vi "ErrorToJSONString.vi"(8 "error in (no error)":errorcluster, 11 "problemJSON":string) -> (0 "error out":errorcluster, 3 "JSON Error string":string)   [LabVIEW 2013]
doc: "Converts an error code into a JSON object, optionally included a properly-quoted copy of the JSON that triggered it. Does not clear the error."
uses:
  <vilib>/Utility/error.llb/DialogType.ctl
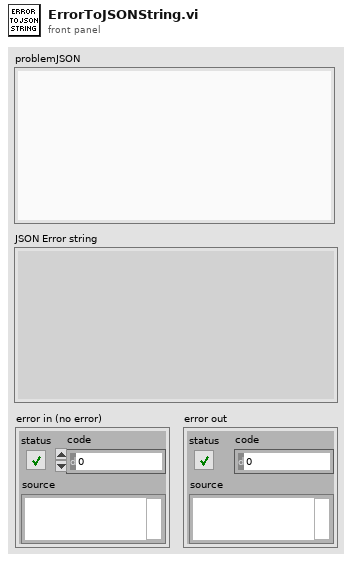
[diagram p1: front panel]
types:
  T1 = cluster{"errorNumber":i32, "errorMessage":string, "problemJSON":string}
  T2 = typedef "DialogType.ctl" = u16
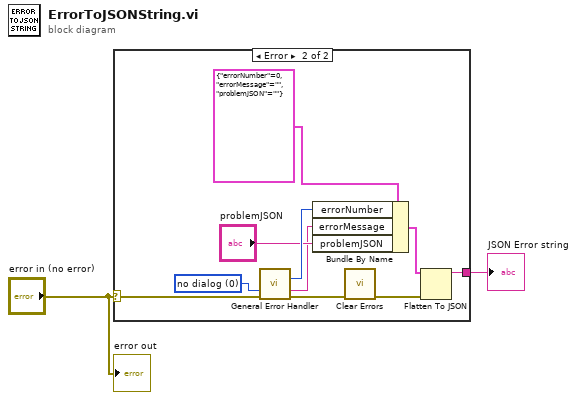
[diagram p0: block diagram]
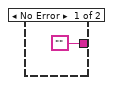
[diagram p2: hidden frame]
diagram:
  n1 = case shown="Error" "error in (no error)" {
    selector: "error in (no error)" -> [_ w5]
    tunnel: ["" w4] -> w1
    frame No Error {
    }
    frame Error {
      w13 = T2 0 items=["no dialog", "OK message", "continue or stop message", "OK message + warnings", "continue/stop + warnings"] ("type of dialog (OK msg:1)")
      n2 = call <vilib>:"General Error Handler.vi"("type of dialog (OK msg:1)"=w13, "error in (no error)"=w5) -> ("code out"=w10:i32, "message"=w7:string, "error out"=w11:errorcluster)  [unwired: 9 in, 2 out]
      n3 = Bundle By Name(cluster=T1 {"errorNumber"=0, "errorMessage"="", "problemJSON"=""}, "errorNumber"=w10, "errorMessage"=w7, "problemJSON"="problemJSON") -> (w9:T1)
      n4 = call <vilib>:"Clear Errors.vi"("error in (no error)"=w11) -> ("error out"=w12:errorcluster)  [unwired: 6 in]
      n5 = Flatten To JSON(anything=w9, error in (no error)=w12) -> (JSON string=w4:string)  [unwired: 1 in, 1 out]
    }
  }
  "JSON Error string" <- w1
  "error out" <- "error in (no error)"
